vi "Initialize Word and Math.vi"(8 "error in (no error)":errorcluster, 9 "MathCAD results":T1, 10 "Slide Refnum":refnum<vi>) -> (0 "error out":errorcluster, 1 "Success":bool)   [LabVIEW 2015, in "AguaClara Library.lvlib"]
uses:
  AguaClara Library.lvlib
  <vilib>/Utility/config.llb/NI_LVConfig.lvlib
  mathcad/Simple/MathCAD cmd.ctl
  Project commands.ctl
  Word cmd.ctl
  <vilib>/Utility/config.llb/Read Key (Boolean).vi
  MathCAD results ref.ctl
panel:
  out "appended path":path
  out "Ini file path":path
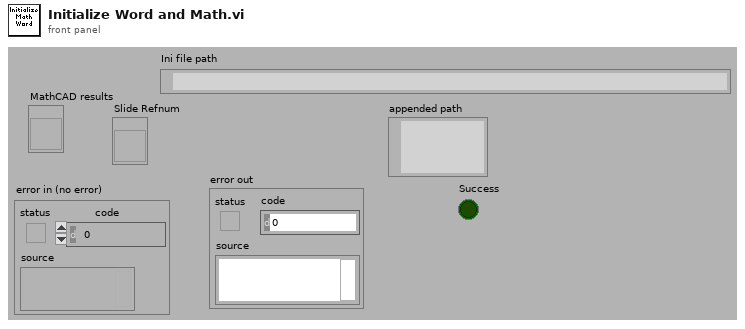
[diagram p1: front panel]
types:
  T1 = typedef "MathCAD results ref.ctl" = refnum<vi>
  T2 = typedef "NI_LVConfig.lvlib/Config Data RefNum.ctl" = refnum<k1>
  T3 = typedef "AguaClara Library.lvlib/Word cmd.ctl" = enum16{"Initialize", "Load User Inputs", "Update Fields", "Replace Variables", "Save pdf", "Close Word"}
  T4 = typedef "MathCAD cmd.ctl" = enum16{"Open App", "Open Worksheet", "Close Worksheet", "Load Variable Ref", "Send Number", "Send Cluster", "Send Array", "Send String", "Calculate", "Get MathCAD data", "Close MathCAD"}
  T5 = typedef "AguaClara Library.lvlib/Project commands.ctl" = enum16{"Load base file", "Load User", "Read paths", "Open Project", "New project", "Edit project", "Delete project", "Mail project", "save design", "open design"}
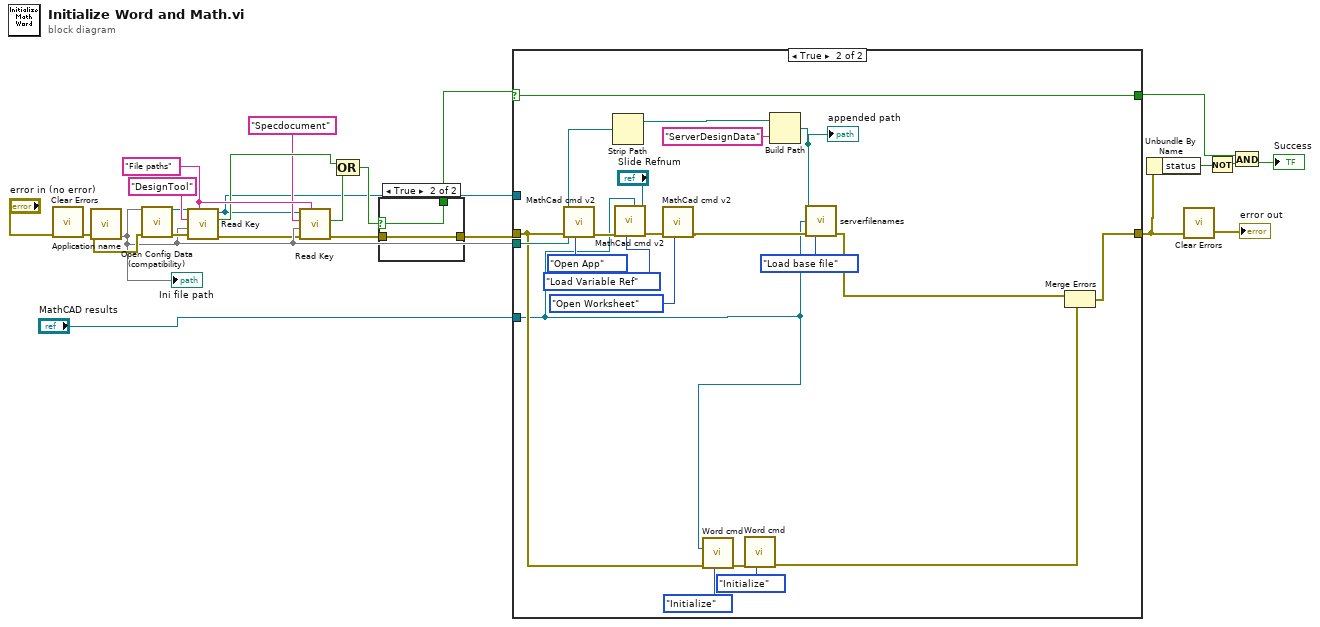
[diagram p0: block diagram]
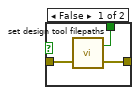
[diagram p2: hidden frame]
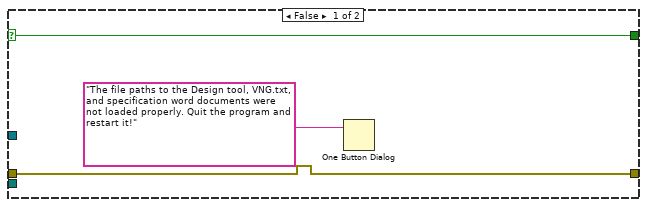
[diagram p3: hidden frame]
diagram:
  w12 = "File paths" ("section")
  n1 = call <vilib>:"Clear Errors.vi"("error in (no error)"="error in (no error)") -> ("error out"=w17:errorcluster)  [unwired: 5 in, 1 out]
  n2 = call "Application name.vi"() -> (0:w8)  [unwired: 4 in, 3 out]
  "Ini file path" <- w8
  n3 = call <vilib>:"Open Config Data (compatibility).vi"("error in (no error)"=w17, "configuration file path"=w8) -> ("error out"=w20:errorcluster, "refnum"=w21:T2)  [unwired: 7 in, 1 out]
  n4 = call-poly <vilib>:"Read Key.vi"("section"=w12, "error in (no error)"=w20, "default value"=w8, "key"="DesignTool", "refnum"=w21) -> ("error out"=w1:errorcluster, "found?"=w10:bool, "refnum out"=w2:T2)  [unwired: 3 in, 1 out]
  n5 = call-poly <vilib>:"Read Key.vi"("section"=w12, "error in (no error)"=w1, "default value"=w8, "key"="Specdocument", "refnum"=w2) -> ("error out"=w7:errorcluster, "found?"=w11:bool)  [unwired: 3 in, 2 out]
  n6 = Compound Arithmetic op=OR(w10, w11) -> (w5:bool)
  n7 = case shown="True" w5 {
    selector: w5 -> [_ w27]
    tunnel: w7 -> [w26 w28]
    tunnel: [w25 w28] -> w6
    tunnel: [w24 w27] -> w4
    frame False {
      n8 = call "set design tool filepaths.vi"("error in (no error)"=w26) -> ("error out"=w25:errorcluster, "Success"=w24:bool)  [unwired: 1 in]
    }
    frame True {
    }
  }
  n9 = case shown="True" w4 {
    selector: w4 -> [w31 w46]
    tunnel: w2 -> [_ _]
    tunnel: [w30 w35] -> w16
    tunnel: w8 -> [_ w47]
    tunnel: "MathCAD results" -> [_ w32]
    tunnel: [w31 w46] -> w3
    tunnel: w6 -> [w30 w34]
    frame False {
      n10 = One Button Dialog(message="The file paths to the Design tool, VNG.txt, and specification word documents were not loaded properly. Quit the program and restart it!") -> ()  [unwired: 1 in, 1 out]
    }
    frame True {
      n11 = call "MathCad cmd v2.vi"("MathCAD cmds"=MathCAD_cmd."Open App", "error in"=w34) -> ("first error out"=w45:errorcluster)  [unwired: 8 in, 1 out]
      n12 = Strip Path(path=w47) -> (stripped path=w48:path)  [unwired: 1 out]
      n13 = call "MathCad cmd v2.vi"("Slide Refnum"="Slide Refnum", "MathCAD variables"=w32, "MathCAD cmds"=MathCAD_cmd."Load Variable Ref", "error in"=w45) -> ("first error out"=w43:errorcluster)  [unwired: 6 in, 1 out]
      n14 = call "MathCad cmd v2.vi"("MathCAD cmds"=MathCAD_cmd."Open Worksheet", "error in"=w43) -> ("first error out"=w33:errorcluster)  [unwired: 8 in, 1 out]
      n15 = call "Word cmd.vi"("Word cmd"=Word_cmd."Initialize", "Error In (no error)"=w34, "Mathcad Output"=w32) -> ("error out"=w39:errorcluster)  [unwired: 7 in, 1 out]
      n16 = call "Word cmd.vi"("Word cmd"=Word_cmd."Initialize", "Error In (no error)"=w39) -> ("error out"=w36:errorcluster)  [unwired: 8 in, 1 out]
      n17 = Build Path(base path=w48, name or relative path="ServerDesignData") -> (appended path=w49:path)
      "appended path" <- w49
      n18 = call "serverfilenames.vi"(5:w49, "MathCAD results"=w32, "error in (no error)"=w33, "Project command"=Project_commands."Load base file") -> ("error out"=w37:errorcluster)  [unwired: 7 in, 4 out]
      n19 = Merge Errors(w37, w36) -> (w35:errorcluster)
    }
  }
  n20 = Unbundle By Name(w16) -> ("status"=w14:bool)
  n21 = call <vilib>:"Clear Errors.vi"("error in (no error)"=w16) -> ("error out"=→"error out":errorcluster)  [unwired: 5 in, 1 out]
  n22 = Not(x=w14) -> (.not. x?=w15:bool)
  n23 = And(x=w3, y=w15) -> (x .and. y?=→"Success":bool)
